vi "fitting_data.vi"(7 "Recorded_Data 2":dbl[][](array[numeric])) -> (0 "R-square":dbl, 1 "intercept":dbl, 2 "slope":dbl, 3 "Recorded_Data 3":dbl[][](array[numeric]))   [LabVIEW 2021]
uses:
  <vilib>/Analysis/6fits.llb/Curve Fitting Criteria.ctl
  <vilib>/Analysis/NI_AALPro.lvlib
panel:
  out "SSE":dbl
  out "subarray 2":dbl[](array[numeric])
  out "subarray":dbl[](array[numeric])
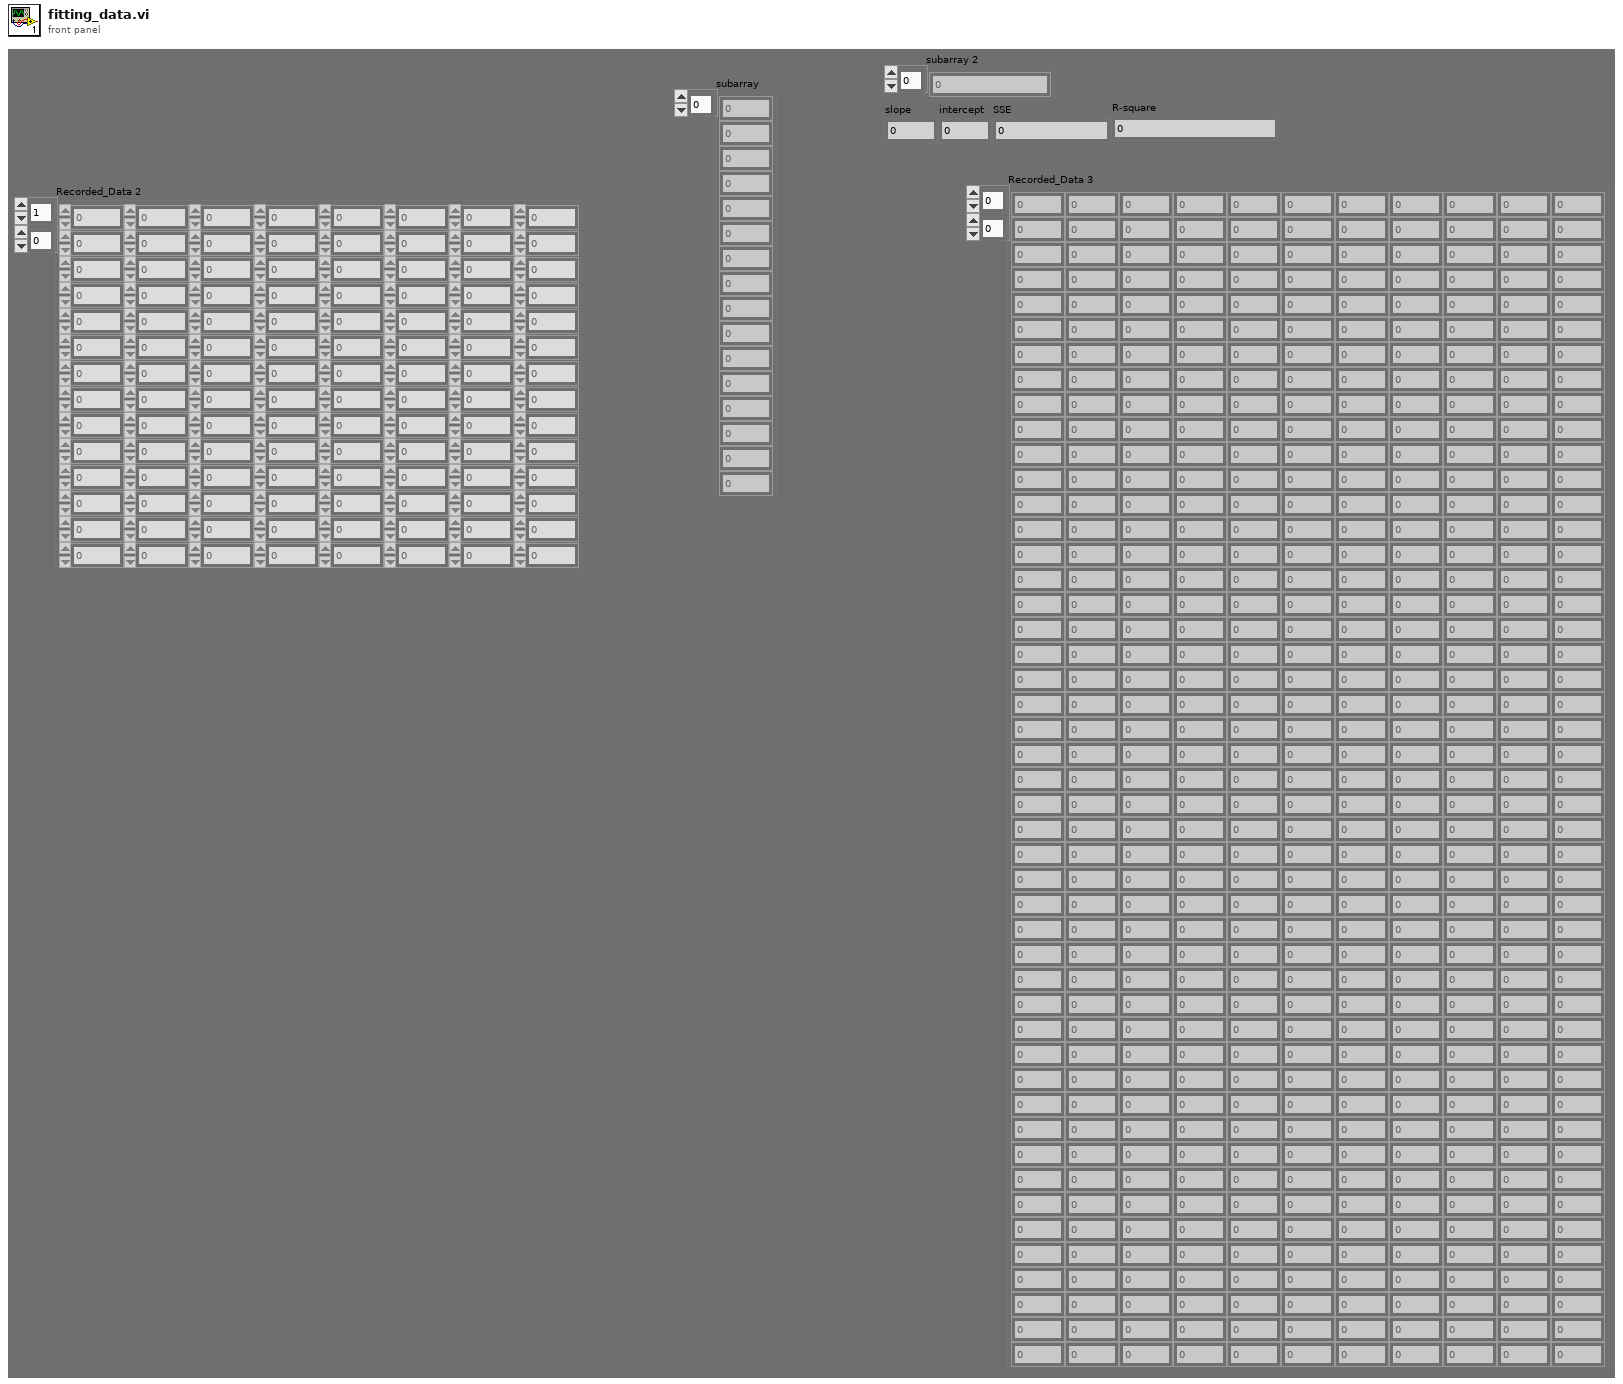
[diagram p1: front panel]
types:
  T1 = typedef "NI_AALPro.lvlib/Curve Fitting Criteria.ctl" = u16
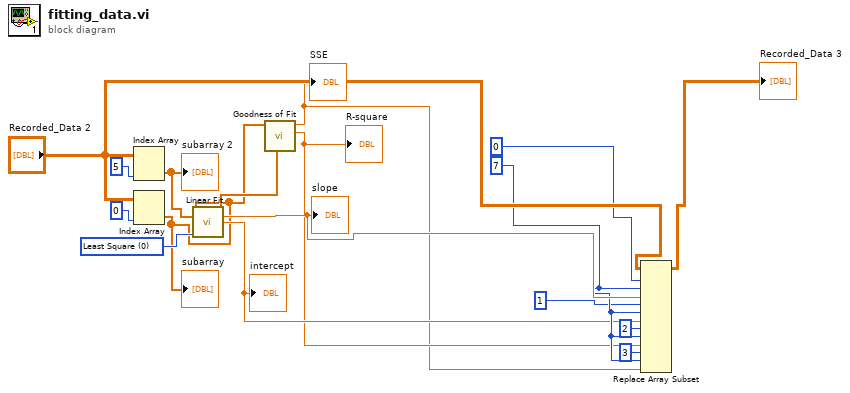
[diagram p0: block diagram]
diagram:
  w9 = 7 ("disabled index (col)")
  w15 = T1 0 items=["Least Square", "Least Absolute Residual", "Bisquare"] ("method")
  n1 = Index Array(array="Recorded_Data 2", index (col)=5 ("disabled index (col)")) -> (element=w2:dbl[])  [unwired: 1 in]
  "subarray 2" <- w2
  n2 = Index Array(array="Recorded_Data 2", index (col)=0 ("disabled index (col)")) -> (element=w1:dbl[])  [unwired: 1 in]
  "subarray" <- w1
  n3 = call <vilib>:"Linear Fit.vi"("Y"=w1, "X"=w2, "method"=w15) -> ("Best Linear Fit"=w14:dbl[], "slope"=w10:dbl, "intercept"=w7:dbl)  [unwired: 8 in, 2 out]
  "slope" <- w10
  "intercept" <- w7
  n4 = call <vilib>:"Goodness of Fit.vi"("Best Fit"=w14, "Y"=w1) -> ("R-square"=w5:dbl, "SSE"=w3:dbl)  [unwired: 6 in, 2 out]
  "SSE" <- w3
  "R-square" <- w5
  n5 = Replace Array Subset(array="Recorded_Data 2", new element #1=w10, index (row) #1=0 ("disabled index (row)"), index (col) #1=w9, new element #2=w7, index (row) #2=1 ("disabled index (row)"), index (col) #2=w9, new element #3=w5, index (row) #3=2 ("disabled index (row)"), index (col) #3=w9, new element #4=w3, index (row) #4=3 ("disabled index (row)"), index (col) #4=w9) -> (→"Recorded_Data 3":dbl[][])
